vi "Position Window on Parent.vi"(8 "error in (no error)":errorcluster, 9 "Offset":T1={"Horizontal"=-1, "Vertical"=-1}, 10 "Parent VI":refnum<vi>, 11 "VI in":refnum<vi>) -> (0 "error out":errorcluster, 3 "VI out":refnum<vi>)   [LabVIEW 2020]
uses:
  <vilib>/Utility/miscctls.llb/LVPoint32TypeDef.ctl
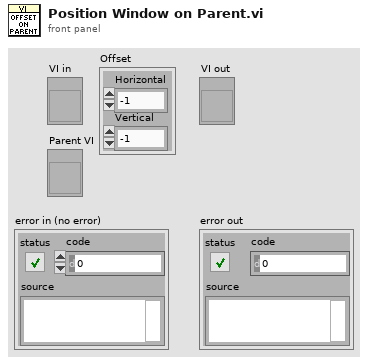
[diagram p1: front panel]
types:
  T1 = typedef "LVPoint32TypeDef.ctl" = cluster{"Horizontal":i32, "Vertical":i32}
  T2 = typedef "LVRectTypeDef.ctl" = cluster{"Left":i16, "Top":i16, "Right":i16, "Bottom":i16}
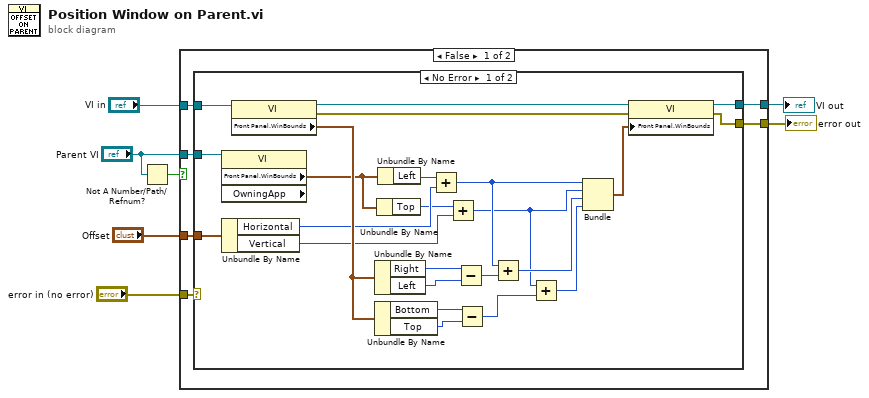
[diagram p0: block diagram]
diagram:
  n1 = Not A Number/Path/Refnum?(number/path/refnum="Parent VI") -> (NaN/Path/Refnum?=w2:bool)
  n2 = case shown="False" w2 {
    tunnel: [w13 w39] -> w7
    tunnel: [w12 w40] -> w6
    tunnel: "error in (no error)" -> [w11 w40]
    tunnel: "VI in" -> [w10 w39]
    tunnel: "Parent VI" -> [w9 _]
    tunnel: "Offset" -> [w8 _]
    frame False {
      n3 = case shown="No Error" w11 {
        tunnel: w10 -> [w37 w38]
        tunnel: [w33 _] -> w12
        tunnel: [w34 w38] -> w13
        tunnel: w9 -> [w24 _]
        tunnel: w8 -> [w22 _]
        frame No Error {
          n4 = property class="VI" props=["Front Panel.WinBounds", "OwningApp"](reference=w24) -> ("Front Panel.WinBounds"=w19:T2)  [unwired: 1 in, 3 out]
          n5 = Unbundle By Name(w22) -> ("Horizontal"=w21:i32, "Vertical"=w17:i32)
          n6 = property class="VI"(reference=w37) -> (reference out=w35:refnum<vi>, error out=w36:errorcluster, "Front Panel.WinBounds"=w26:T2)  [unwired: 1 in]
          n7 = Unbundle By Name(w26) -> ("Right"=w32:i16, "Left"=w31:i16)
          n8 = Unbundle By Name(w26) -> ("Bottom"=w30:i16, "Top"=w29:i16)
          n9 = Unbundle By Name(w19) -> ("Top"=w18:i16)
          n10 = Unbundle By Name(w19) -> ("Left"=w23:i16)
          n11 = Add(x=w23, y=w21) -> (x+y=w20:i32)
          n12 = Add(x=w18, y=w17) -> (x+y=w16:i32)
          n13 = Subtract(x=w32, y=w31) -> (x-y=w28:i16)
          n14 = Subtract(x=w30, y=w29) -> (x-y=w15:i16)
          n15 = Add(x=w20, y=w28) -> (x+y=w27:i32)
          n16 = Add(x=w16, y=w15) -> (x+y=w14:i32)
          n17 = Bundle(w20, w16, w27, w14) -> (w25:cluster{i32, i32, i32, i32})  [unwired: 1 in]
          n18 = property class="VI"(reference=w35, error in=w36, "Front Panel.WinBounds"=w25) -> (reference out=w34:refnum<vi>, error out=w33:errorcluster)
        }
        frame Error {
        }
      }
    }
    frame True {
    }
  }
  "VI out" <- w7
  "error out" <- w6
